vi "Teleop.vi"(10 "Match Info":T3={"Autonomous Elapsed Seconds"=0.0, "TeleOp Elapsed Seconds"=0.0, "Disabled Elapsed Seconds"=0.0, "Visited Autonomous"=FALSE, "Visited TeleOp"=FALSE, "Visited Disabled"=FALSE, "Autonomous Settings"={"Autonomous Style"=enum."Independent", "VI Refnum"=refnum}}, 11 "Call Context":T4) -> ()   [LabVIEW 2016]
doc: "This VI is called for each TeleOp packet received from the DS where the robot is not disabled. It is often used to read from the joysticks and update I/O or to update setpoints for timed control loops. It should complete and return within 20 milliseconds or it may miss DS packets."
uses:
  <vilib>/Rock Robotics/WPI/DriverStation/WPI_DriverStationDerivedRobotMode.ctl
  <vilib>/Rock Robotics/WPI/DriverStation/WPI_DriverStationMatch Info.ctl
  <vilib>/Rock Robotics/WPI/ThirdParty/CanMotor/TalonSRX/WPI_CANTalonSRX_APIFeedbackSelect.ctl
  <vilib>/Rock Robotics/WPI/ThirdParty/CanMotor/TalonSRX/WPI_CANTalonSRX_APIControlMode.ctl
  <vilib>/addons/control/pid/pid.llb/PID (DBL).vi
  <vilib>/addons/control/pid/NI_PID_pid.lvlib
panel:
  in  "Use LV PID":bool
  in  "PID gains":T1={"proportional gain (Kc)"=0.0, "integral time (Ti, min)"=0.01, "derivative time (Td, min)"=0.0} {"derivative time (Td, min)" format="%.3f"; "integral time (Ti, min)" format="%.3f"; "proportional gain (Kc)" format="%.3f"}
  in  "Feeder %":dbl(slide)=-1.0 scale=-1.0..1.0
  in  "Number of iterations":i32=10
  in  "Reverse Closed-Loop Output":bool
  in  "Reverse Feedback Sensor":bool
  in  "Hopper %":dbl(slide)=1.0 scale=0.0..1.0
  in  "Feedback Reference Shooter":T2=enum."CTR Magnetic Enc (Relative)"
  out "Plotted Speed":cluster{"x":dbl, "Sensor Velocity":dbl}[](graph)
  in  "% output Shooter":dbl(slide) scale=0.0..1.0
  in  "Target RPM":dbl(slide)=3150.0 scale=-200.0..5000.0
  in  "Use Speed as control?":bool=TRUE
  out "SensorPosRotations":dbl
  out "Motor output Plot":cluster{"Applied Throttle":dbl}(graph)
  out "Target RPM":dbl
  out "SensorRPM Velocity RPM":dbl
  in  "Ramp Rate":dbl=1.2
  in  "I Zone":dbl
  in  "F":dbl
  in  "D":dbl=0.0002
  in  "I":dbl=0.0001
  in  "P":dbl=0.2425
  out "Applied Output":dbl
  out "Speed Closed Loop Plots":cluster{dbl, "Sensor Velocity":dbl}(graph)
  # "was max of 5000"
  # "Use the Left Y-axis on Logitech Gamepad.\n\nVelocityNativeUnits = Change In Sensor / 100mS\nalso\nVelocityNativeUnits = RPM / 600 * SensorUnitsPerRotation\n\nFgain = 100% X 1023 / VelocityNativeUnits , \n       where VelocityNativeUnits  is measured at 100% throttle\n\nMag Encoder has 4096 units per rotation.\n\nExample: VelocityRPM is 10198 at 100% throttle\n                 => VelocityNativeUnits = (10198 / 600 * 4096) = 69618\n                 => Fgain = (1023 / 69618)  = 0.01469"
  # "was 6.8266667"
  # "ran well \nat about\n.625"
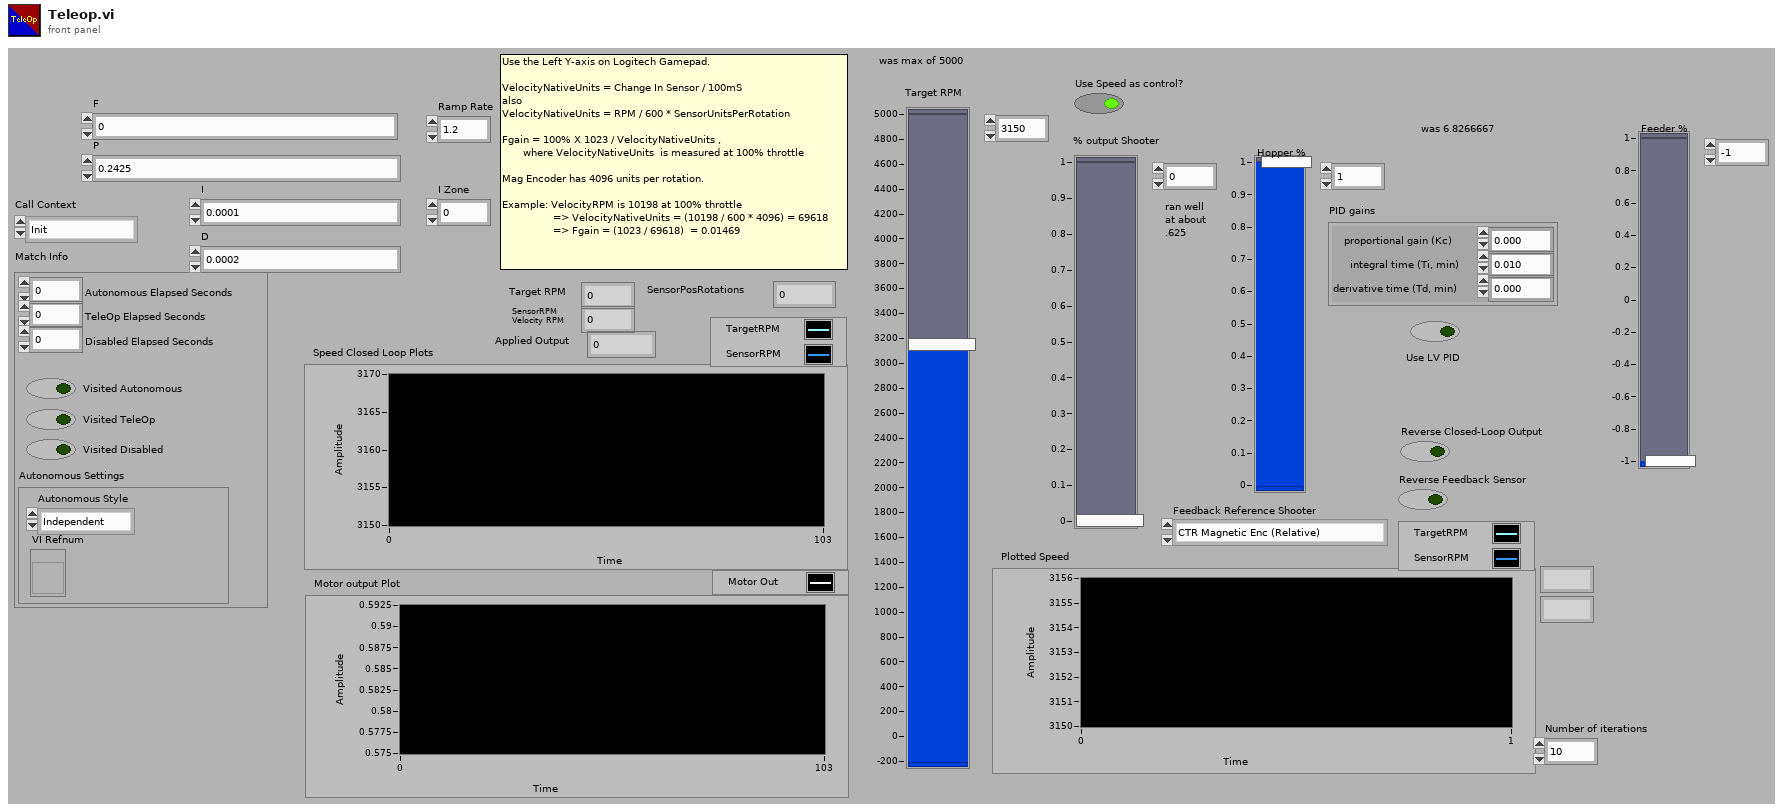
[diagram p1: front panel]
types:
  T1 = cluster{"proportional gain (Kc)":dbl, "integral time (Ti, min)":dbl, "derivative time (Td, min)":dbl}
  T2 = typedef "WPI_CANTalonSRX_APIFeedbackSelect.ctl" = enum16{"Digital Quadrature Encoder", "Analog Potentiometer", "Analog Encoder", "Count on Quad-A (Rising-Edge)", "Count on Quad-A (Falling-Edge)", "CTR Magnetic Enc (Absolute)", "CTR Magnetic Enc (Relative)", "Pulse Width"}
  T3 = typedef "WPI_DriverStationMatch Info.ctl" = cluster{"Autonomous Elapsed Seconds":dbl, "TeleOp Elapsed Seconds":dbl, "Disabled Elapsed Seconds":dbl, "Visited Autonomous":bool, "Visited TeleOp":bool, "Visited Disabled":bool, "Autonomous Settings":cluster{"Autonomous Style":enum16{"Iterative", "Independent"}, "VI Refnum":refnum<vi>}}
  T4 = typedef "WPI_DriverStationDerivedRobotMode.ctl" = enum16{"Init", "Execute", "Stop"}
  T5 = typedef "WPI_CANTalonSRX_APIControlMode.ctl" = enum8{"Percent VBus", "Speed", "Position", "Slave", "Unchanged / Invalid", "Voltage Compensation", "Current", "Motion Profile", "Motion Magic"}
  T6 = typedef "WPI_MotorControlDeviceRef.ctl" = cluster{"DeviceStatus":errorcluster, "Type":T7, "PWM":cluster{"PWM Channel":T8, "DeadBand":T9}, "CAN":cluster{"Device Number":u8, "SetOutput VI Ref":variant, "GetOutput VI Ref":variant, "Enable VI Ref":variant, "Disable VI Ref":variant, "Data":variant}, "Invert":bool}
  T7 = typedef "WPI_MotorControlType.ctl" = enum16{"PWM", "CAN"}
  T8 = typedef "FPGA_DIOPWMChannel.ctl" = enum8{"PWM 0", "PWM 1", "PWM 2", "PWM 3", "PWM 4", "PWM 5", "PWM 6", "PWM 7", "PWM 8", "PWM 9", "PWM MXP 0", "PWM MXP 1", "PWM MXP 2", "PWM MXP 3", "PWM MXP 4", "PWM MXP 5", "PWM MXP 6", "PWM MXP 7", "PWM MXP 8", "PWM MXP 9", "Invalid"}
  T9 = typedef "WPI_PWMDeadband.ctl" = cluster{"Name":string, "maxPositivePwm":i32, "minPositivePwm":i32, "centerPwm":i32, "maxNegativePwm":i32, "minNegativePwm":i32, "angularRange":u16}
  T10 = typedef "WPI_CANTalonSRX_GlobalStatus.ctl" = cluster{"Applied Throttle":dbl, "Module Enabled":bool, "CAN Error":errorcluster, "Closed Loop Error":dbl, "Forward Limit Switch Closed":bool, "Reverse Limit Switch Closed":bool, "Sensor Position":dbl, "Sensor Velocity":dbl, "Current":dbl, "Sticky Fault - Over Temp":bool, "Sticky Fault - Under Voltage":bool, "Sticky Fault - Forward Limit":bool, "Sticky Fault - Reverse Limit":bool, "Sticky Fault - Forward Soft Limit":bool, "Sticky Fault - Reverse Soft Limit":bool, "Brake is Enabled":bool, "Encoder Position":dbl, "Encoder Velocity":dbl, "Encoder Index Count":dbl, "Encoder A Pin State":bool, "Encoder B Pin State":bool, "Encoder Index Pin State":bool, "Analog In":dbl, "Analog In Velocity":dbl, "Temperature (C)":dbl, "Battery Voltage":dbl, "Control 5 Is Supported":bool, "Current Profile Slot Select":dbl, "Pos Div 8":bool, "Vel Div 4":bool, "Pulse Width Position":i32, "Pulse Width Velocity":i32, "Pulse Width Rise To Rise (us)":i32, "Pulse Width Rise To Fall (us)":i32, "Mot Prof Active Is Under Run":bool, "Mot Prof Active Has Under Run":bool, "Mot Prof Active Is Last":bool, "Mot Prof Active Velocity Only":bool, "Mot Prof Active Is Valid":bool, "Mot Prof Buffer Is Full":bool, "Mot Prof Active Profile Slot Select":i32, "Mot Prof NextID":i32, "Mot Prof Count":i32, "Mot Prof Active Velocity":dbl, "Mot Prof Active Position":dbl, "Mot Prof Output Enable":i32}
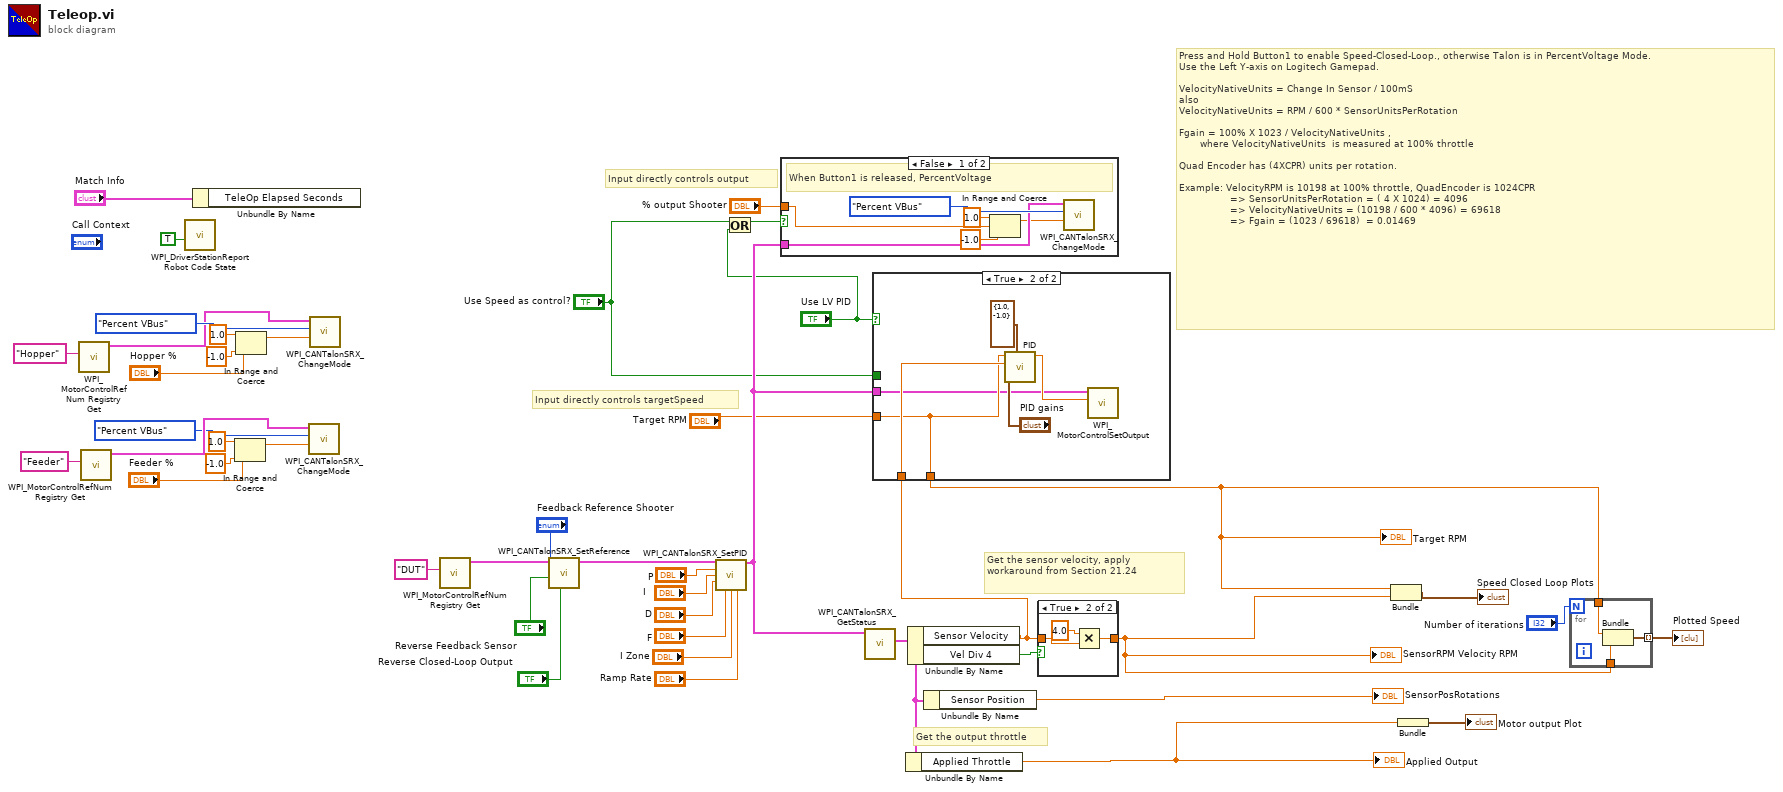
[diagram p0: block diagram]
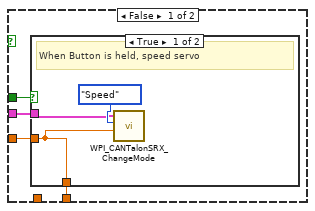
[diagram p2: hidden frame]
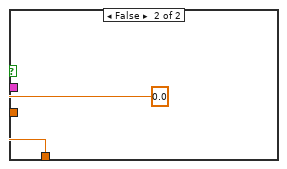
[diagram p3: hidden frame]
diagram:
  # "Press and Hold Button1 to enable Speed-Closed-Loop., otherwise Talon is in PercentVoltage Mode.  \nUse the Left Y-axis on Logitech Gamepad.\n\nVelocityNativeUnits = Change In Sensor / 100mS\nalso\nVelocityNativeUnits = RPM / 600 * SensorUnitsPerRotation\n\nFgain = 100% X 1023 / VelocityNativeUnits , \n       where VelocityNativeUnits  is measured at 100% throttle\n\nQuad Encoder has (4XCPR) units per rotation.\n\nExample: VelocityRPM is 10198 at 100% throttle, QuadEncoder is 1024CPR\n                 => SensorUnitsPerRotation = ( 4 X 1024) = 4096\n                 => VelocityNativeUnits = (10198 / 600 * 4096) = 69618\n                 => Fgain = (1023 / 69618)  = 0.01469"
  # "Get the output throttle"
  # "Get the sensor velocity, apply workaround from Section 21.24"
  # "Input directly controls targetSpeed"
  # "Input directly controls output"
  n1 = call <vilib>:"WPI_MotorControlRefNum Registry Get.vi"("refnum name"="Hopper") -> ("MotorControlDevRef"=w26:T6)  [unwired: 9 in, 1 out]
  n2 = call <vilib>:"WPI_MotorControlRefNum Registry Get.vi"("refnum name"="Feeder") -> ("MotorControlDevRef"=w15:T6)  [unwired: 9 in, 1 out]
  n3 = call <vilib>:"WPI_DriverStationReport Robot Code State.vi"("TeleOp"=TRUE ("Autonomous")) -> ()  [unwired: 10 in, 1 out]
  n4 = Unbundle By Name("Match Info") -> ()  [unwired: 1 out]
  n5 = In Range and Coerce(upper limit=1.0, x="Feeder %", lower limit=-1.0) -> (coerced(x)=w17:dbl)  [unwired: 1 out]
  n6 = In Range and Coerce(upper limit=1.0, x="Hopper %", lower limit=-1.0) -> (coerced(x)=w24:dbl)  [unwired: 1 out]
  n7 = call <vilib>:"WPI_CANTalonSRX_ChangeMode.vi"("Output"=w17, "Control Mode"=WPI_CANTalonSRX_APIControlMode."Percent VBus", "CAN Talon SRX Ref"=w15) -> ()  [unwired: 7 in, 2 out]
  n8 = call <vilib>:"WPI_CANTalonSRX_ChangeMode.vi"("Output"=w24, "Control Mode"=WPI_CANTalonSRX_APIControlMode."Percent VBus", "CAN Talon SRX Ref"=w26) -> ()  [unwired: 7 in, 2 out]
  n9 = call <vilib>:"WPI_MotorControlRefNum Registry Get.vi"("refnum name"="DUT") -> ("MotorControlDevRef"=w40:T6)  [unwired: 9 in, 1 out]
  n10 = call <vilib>:"WPI_CANTalonSRX_SetReference.vi"("Reverse Closed-Loop Output"="Reverse Closed-Loop Output", "Reverse Feedback Sensor"="Reverse Feedback Sensor", "Feedback Reference"="Feedback Reference Shooter", "CAN Talon SRX Ref"=w40) -> ("CAN Talon SRX Ref"=w39:T6)  [unwired: 6 in, 1 out]
  n11 = call <vilib>:"WPI_CANTalonSRX_SetPID.vi"("CAN Talon SRX Ref"=w39, "P"="P", "I"="I", "D"="D", "F"="F", "I Zone"="I Zone", "Ramp Rate"="Ramp Rate") -> ("CAN Talon SRX Ref"=w35:T6)  [unwired: 7 in, 1 out]
  n12 = Or(x="Use Speed as control?", y="Use LV PID") -> (x .or. y?=w4:bool)
  n13 = case shown="False" w4 {
    tunnel: "% output Shooter" -> [w49 _]
    tunnel: w35 -> [w50 _]
    frame False {
      # "When Button1 is released, PercentVoltage"
      n14 = In Range and Coerce(upper limit=1.0, x=w49, lower limit=-1.0) -> (coerced(x)=w46:dbl)  [unwired: 1 out]
      n15 = call <vilib>:"WPI_CANTalonSRX_ChangeMode.vi"("Output"=w46, "Control Mode"=WPI_CANTalonSRX_APIControlMode."Percent VBus", "CAN Talon SRX Ref"=w50) -> ()  [unwired: 7 in, 2 out]
    }
    frame True {
    }
  }
  n16 = call <vilib>:"WPI_CANTalonSRX_GetStatus.vi"("CAN Talon SRX Ref"=w35) -> ("Talon SRX Status"=w37:T10)  [unwired: 8 in, 2 out]
  n17 = Unbundle By Name(w37) -> ("Applied Throttle"=w33:dbl)
  "Applied Output" <- w33
  n18 = Unbundle By Name(w37) -> ("Sensor Velocity"=w5:dbl, "Vel Div 4"=w41:bool)
  n19 = case shown="True" "Use LV PID" {
    tunnel: w35 -> [w55 w60]
    tunnel: "Use Speed as control?" -> [w54 _]
    tunnel: "Target RPM" -> [w53 w61]
    tunnel: [w52 w61] -> w2
    tunnel: w5 -> [_ w62]
    frame False {
      n20 = case shown="True" w54 {
        tunnel: w53 -> [w56 _]
        tunnel: w55 -> [w57 _]
        tunnel: [w56 0.0 ("x")] -> w52
        frame True {
          # "When Button is held, speed servo"
          n21 = call <vilib>:"WPI_CANTalonSRX_ChangeMode.vi"("Output"=w56, "Control Mode"=WPI_CANTalonSRX_APIControlMode."Speed", "CAN Talon SRX Ref"=w57) -> ()  [unwired: 7 in, 2 out]
        }
        frame False {
        }
      }
    }
    frame True {
      n22 = call-poly <vilib>:"PID.vi"("output range"=cluster{"output high":dbl, "output low":dbl} {"output high"=1.0, "output low"=-1.0}, "PID gains"="PID gains", "process variable"=w62, "setpoint"=w61) -> ("output"=w65:dbl)  [unwired: 6 in, 1 out]
      n23 = call <vilib>:"WPI_MotorControlSetOutput.vi"("Output"=w65, "MotorControlDevRef"=w60) -> ()  [unwired: 7 in, 3 out]
    }
  }
  "Target RPM" <- w2
  n24 = Unbundle By Name(w37) -> ("Sensor Position"=→"SensorPosRotations":dbl)
  n25 = case shown="True" w41 {
    tunnel: [w66 w68] -> w1
    tunnel: w5 -> [w66 w67]
    frame False {
    }
    frame True {
      n26 = Multiply(x=4.0, y=w67) -> (x*y=w68:dbl)
    }
  }
  "SensorRPM Velocity RPM" <- w1
  n27 = Bundle("Target RPM"=w2, "Sensor Velocity"=w1) -> (→"Speed Closed Loop Plots":cluster{"Target RPM":dbl, "Sensor Velocity":dbl})  [unwired: 1 in]
  n28 = Bundle("Applied Throttle"=w33) -> (→"Motor output Plot":cluster{"Applied Throttle":dbl})  [unwired: 1 in]
  n29 = for {
    N: "Number of iterations" -> [_]
    tunnel: w2 -> [w72]
    tunnel: w1 -> [w71]
    tunnel: [w70] -> w19 mode=indexing
    n30 = Bundle("Target RPM"=w72, "Sensor Velocity"=w71) -> (w70:cluster{"Target RPM":dbl, "Sensor Velocity":dbl})  [unwired: 1 in]
  }
  "Plotted Speed" <- w19
